vi "VGD ECL AHMI PF SubVI03.vi"(0 "FRONTAL":T2, 1 "SUPERIOR":T2, 2 "pixmap COLOR":u32[][](array[numeric]), 3 "pixmap GF":u32[][](array[numeric]), 4 "pixmap GS":u32[][](array[numeric]), 5 "error in":errorcluster, 7 "Color":u32(colorbox)=16711680, 9 "Factor diezmado":i32) -> (14 "FRONTAL":T2, 15 "SUPERIOR":T2, 16 "Rfront":T1, 17 "Rsup":T1, 19 "error out":errorcluster)   [LabVIEW 2020]
uses:
  <vilib>/vision/Image Controls.llb/IMAQ Image.ctl
  <vilib>/ptbypt/NI_PtbyPt.lvlib
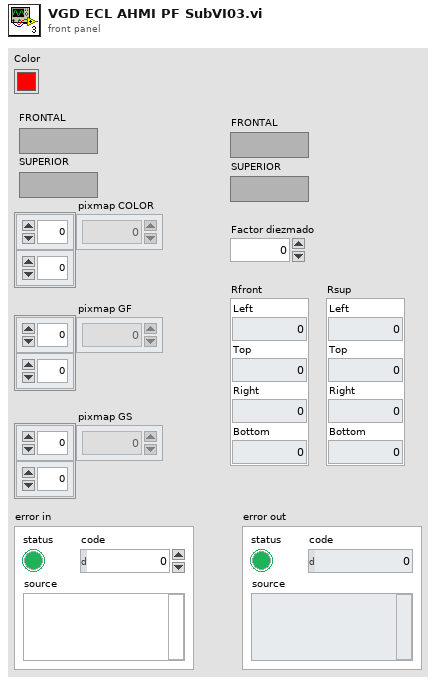
[diagram p1: front panel]
types:
  T1 = cluster{"Left":i32, "Top":i32, "Right":i32, "Bottom":i32}
  T2 = typedef "IMAQ Image.ctl" = refnum<image>
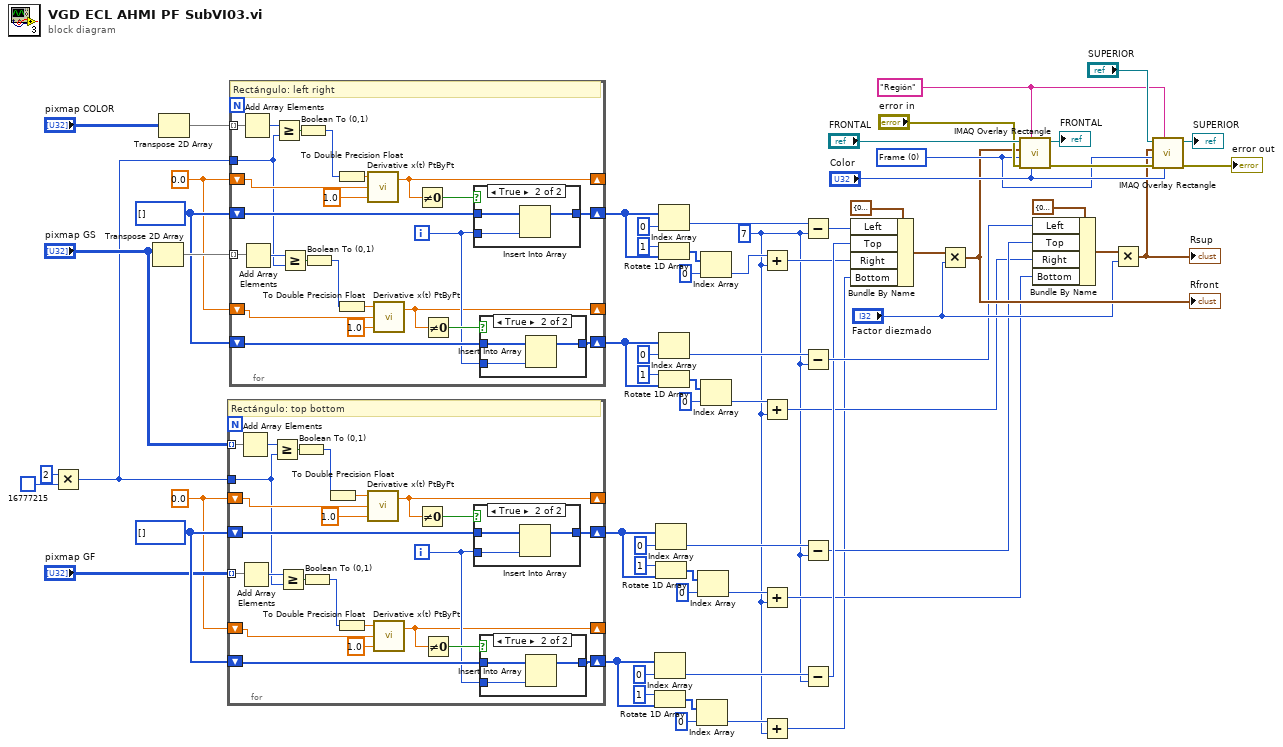
[diagram p0: block diagram]
diagram:
  w3 = 7 ("y")
  w49 = "Región" ("Group")
  w45 = u32 0 items=["Frame", "Fill", "Highlight"] ("Drawing Mode (Frame)")
  w62 = i32[] []
  w21 = 0.0 ("dx/dt")
  w63 = i32[] []
  w20 = 0.0 ("dx/dt")
  n1 = Multiply(x=u32 2, y=u32 16777215) -> (x*y=w1:u32)
  n2 = Transpose 2D Array(2D array="pixmap GS") -> (transposed array=w64:u32[][])
  n3 = Transpose 2D Array(2D array="pixmap COLOR") -> (transposed array=w65:u32[][])
  n4 = for {
    tunnel: "pixmap GS" -> [w90] mode=indexing
    tunnel: w1 -> [w75]
    shift-right: [w68] -> _
    shift-left: w21 -> [w86]
    shift-right: [w82] -> w27
    shift-left: w62 -> [w83]
    tunnel: "pixmap GF" -> [w76] mode=indexing
    shift-right: [w71] -> w22
    shift-left: w62 -> [w74]
    shift-right: [w67] -> _
    shift-left: w21 -> [w72]
    i -> [w73]
    # "Rectángulo: top bottom"
    n5 = Add Array Elements(numeric array=w90) -> (sum=w89:u32)
    n6 = Add Array Elements(numeric array=w76) -> (sum=w77:u32)
    n7 = Greater Or Equal?(x=w89, y=w75) -> (x >= y?=w88:bool)
    n8 = Greater Or Equal?(x=w77, y=w75) -> (x >= y?=w78:bool)
    n9 = Boolean To (0,1)(Boolean=w88) -> (0, 1=w87:i16)
    n10 = Boolean To (0,1)(Boolean=w78) -> (0, 1=w79:i16)
    n11 = To Double Precision Float(number=w87) -> (double precision float=w70:dbl)
    n12 = To Double Precision Float(number=w79) -> (double precision float=w69:dbl)
    n13 = call <vilib>:"Derivative x(t) PtByPt.vi"("dt"=1.0, "initial condition"=w86, "x"=w70) -> ("dx/dt"=w68:dbl)  [unwired: 1 in, 1 out]
    n14 = call <vilib>:"Derivative x(t) PtByPt.vi"("dt"=1.0, "initial condition"=w72, "x"=w69) -> ("dx/dt"=w67:dbl)  [unwired: 1 in, 1 out]
    n15 = Not Equal To 0?(x=w68) -> (x != 0?=w84:bool)
    n16 = Not Equal To 0?(x=w67) -> (x != 0?=w81:bool)
    n17 = case shown="True" w84 {
      tunnel: w83 -> [w95 w98]
      tunnel: w73 -> [_ w97]
      tunnel: [w95 w96] -> w82
      frame False {
      }
      frame True {
        n18 = Insert Into Array(array=w98, new element=w97) -> (w96:i32[])  [unwired: 1 in]
      }
    }
    n19 = case shown="True" w81 {
      tunnel: w74 -> [w91 w94]
      tunnel: w73 -> [_ w93]
      tunnel: [w91 w92] -> w71
      frame False {
      }
      frame True {
        n20 = Insert Into Array(array=w94, new element=w93) -> (w92:i32[])  [unwired: 1 in]
      }
    }
  }
  n21 = for {
    tunnel: w65 -> [w122] mode=indexing
    tunnel: w1 -> [w106]
    shift-right: [w114] -> _
    shift-left: w20 -> [w118]
    shift-right: [w113] -> w40
    shift-left: w63 -> [w115]
    tunnel: w64 -> [w107] mode=indexing
    shift-right: [w101] -> w32
    shift-left: w63 -> [w105]
    shift-right: [w103] -> _
    shift-left: w20 -> [w102]
    i -> [w104]
    # "Rectángulo: left right"
    n22 = Add Array Elements(numeric array=w122) -> (sum=w121:u32)
    n23 = Add Array Elements(numeric array=w107) -> (sum=w108:u32)
    n24 = Greater Or Equal?(x=w121, y=w106) -> (x >= y?=w120:bool)
    n25 = Greater Or Equal?(x=w108, y=w106) -> (x >= y?=w109:bool)
    n26 = Boolean To (0,1)(Boolean=w120) -> (0, 1=w119:i16)
    n27 = Boolean To (0,1)(Boolean=w109) -> (0, 1=w110:i16)
    n28 = To Double Precision Float(number=w119) -> (double precision float=w100:dbl)
    n29 = To Double Precision Float(number=w110) -> (double precision float=w99:dbl)
    n30 = call <vilib>:"Derivative x(t) PtByPt.vi"("dt"=1.0, "initial condition"=w118, "x"=w100) -> ("dx/dt"=w114:dbl)  [unwired: 1 in, 1 out]
    n31 = call <vilib>:"Derivative x(t) PtByPt.vi"("dt"=1.0, "initial condition"=w102, "x"=w99) -> ("dx/dt"=w103:dbl)  [unwired: 1 in, 1 out]
    n32 = Not Equal To 0?(x=w114) -> (x != 0?=w116:bool)
    n33 = Not Equal To 0?(x=w103) -> (x != 0?=w112:bool)
    n34 = case shown="True" w116 {
      tunnel: w115 -> [w127 w130]
      tunnel: w104 -> [_ w129]
      tunnel: [w127 w128] -> w113
      frame False {
      }
      frame True {
        n35 = Insert Into Array(array=w130, new element=w129) -> (w128:i32[])  [unwired: 1 in]
      }
    }
    n36 = case shown="True" w112 {
      tunnel: w105 -> [w123 w126]
      tunnel: w104 -> [_ w125]
      tunnel: [w123 w124] -> w101
      frame False {
      }
      frame True {
        n37 = Insert Into Array(array=w126, new element=w125) -> (w124:i32[])  [unwired: 1 in]
      }
    }
  }
  n38 = Index Array(array=w22, index=0) -> (element=w15:i32)
  n39 = Rotate 1D Array(1:w22, 2:1 ("n")) -> (0:w26:i32[])
  n40 = Index Array(array=w27, index=0) -> (element=w13:i32)
  n41 = Rotate 1D Array(1:w27, 2:1 ("n")) -> (0:w28:i32[])
  n42 = Index Array(array=w40, index=0) -> (element=w18:i32)
  n43 = Rotate 1D Array(1:w40, 2:1 ("n")) -> (0:w37:i32[])
  n44 = Index Array(array=w32, index=0) -> (element=w17:i32)
  n45 = Rotate 1D Array(1:w32, 2:1 ("n")) -> (0:w36:i32[])
  n46 = Index Array(array=w26, index=0) -> (element=w5:i32)
  n47 = Index Array(array=w28, index=0) -> (element=w7:i32)
  n48 = Index Array(array=w37, index=0) -> (element=w10:i32)
  n49 = Index Array(array=w36, index=0) -> (element=w9:i32)
  n50 = Add(x=w10, y=w3) -> (x+y=w11:i32)
  n51 = Add(x=w9, y=w3) -> (x+y=w8:i32)
  n52 = Add(x=w7, y=w3) -> (x+y=w6:i32)
  n53 = Add(x=w5, y=w3) -> (x+y=w4:i32)
  n54 = Subtract(x=w18, y=w3) -> (x-y=w19:i32)
  n55 = Subtract(x=w17, y=w3) -> (x-y=w16:i32)
  n56 = Subtract(x=w13, y=w3) -> (x-y=w12:i32)
  n57 = Subtract(x=w15, y=w3) -> (x-y=w14:i32)
  n58 = Bundle By Name(cluster=T1 {"Left"=0, "Top"=0, "Right"=0, "Bottom"=0} ("Rectangle"), "Left"=w19, "Top"=w14, "Right"=w11, "Bottom"=w4) -> (w55:T1)
  n59 = Multiply(x=w55, y="Factor diezmado") -> (x*y=w43:T1)
  "Rfront" <- w43
  n60 = call "IMAQ Overlay Rectangle"("Color"="Color", "Group"=w49, "error in (no error)"="error in", "Drawing Mode (Frame)"=w45, "Rectangle"=w43, "Image"="FRONTAL") -> ("error out"=w52:errorcluster, "Image Out"=→"FRONTAL":T2)  [unwired: 4 in]
  n61 = Bundle By Name(cluster=T1 {"Left"=0, "Top"=0, "Right"=0, "Bottom"=0} ("Rectangle"), "Left"=w16, "Top"=w12, "Right"=w8, "Bottom"=w6) -> (w47:T1)
  n62 = Multiply(x=w47, y="Factor diezmado") -> (x*y=w42:T1)
  "Rsup" <- w42
  n63 = call "IMAQ Overlay Rectangle"("Color"="Color", "Group"=w49, "error in (no error)"=w52, "Drawing Mode (Frame)"=w45, "Rectangle"=w42, "Image"="SUPERIOR") -> ("error out"=→"error out":errorcluster, "Image Out"=→"SUPERIOR":T2)  [unwired: 4 in]
